vi "OTP - Determine bits.vi"(7 "Specification":T1={"Cmin (fF)"=500.0, "Cmin tolerance (%)"=10.0, "Cmax (fF)"=3460.0, "Cmax tolerance (%)"=1.38, "States"=32}, 8 "Cmax measured (fF)":dbl, 9 "Cmin measured (fF)":dbl=595.842, 10 "dCap (fF)":dbl[](array[numeric])=[216.58100000000002, 226.95699999999997, 198.55200000000005, 220.50100000000006, 199.26699999999997, 240.08200000000002, 67.724, 255.87100000000007, 215.32300000000004, 199.00000000000006, 230.48900000000006, 201.30599999999998, 137.042, 42.55399999999998], 11 "Register 2 & 3 (hex)":string[][](array[string])=[["1", "0"]]) -> (1 "Target values (fF)":dbl[](array[numeric]), 2 "Measured values (fF)":dbl[](array[numeric]), 3 "Register 2 & 3 (hex)":string[][](array[string]))   [LabVIEW 2020]
panel:
  out "Error":dbl[](graph)
  out "Measured vs. Target error (%)":dbl[](array[numeric])
  out "System Waveform Graph":dbl[][](graph)
  out "max value":dbl
  out "min value":dbl
  out "Setting indices":dbl[](array[numeric])
  out "Setting beams":bool[][](array[boolean])
  out "Measured-Target (fF)":dbl[](array[numeric])
  out "All comb. meas (fF)":dbl[](array[numeric])
  out "Target step (fF)":dbl
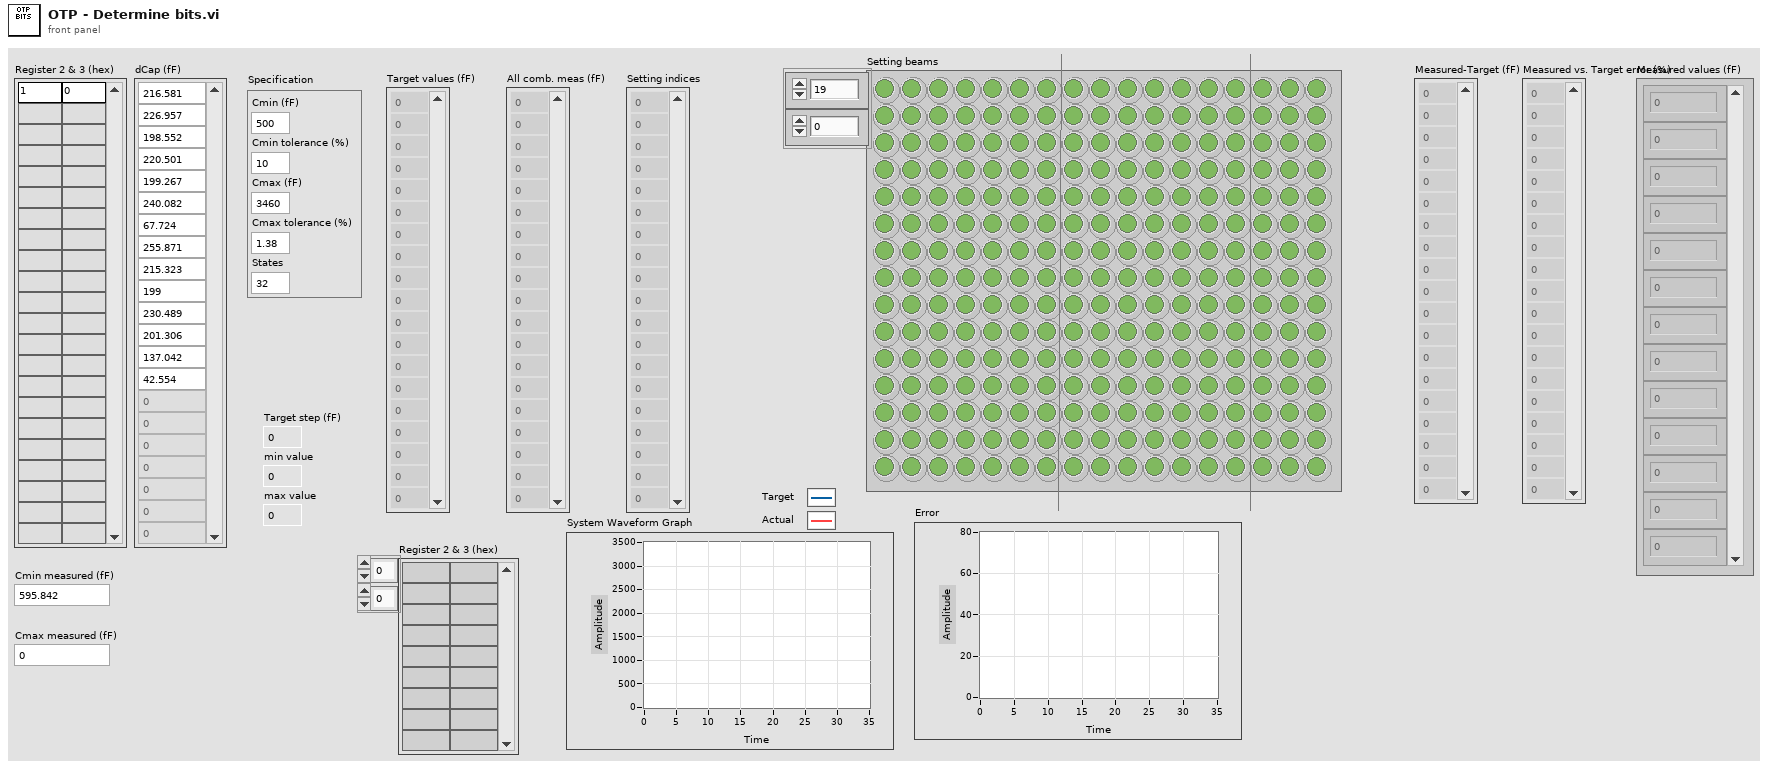
[diagram p1: front panel]
types:
  T1 = cluster{"Cmin (fF)":dbl, "Cmin tolerance (%)":dbl, "Cmax (fF)":dbl, "Cmax tolerance (%)":dbl, "States":i32}
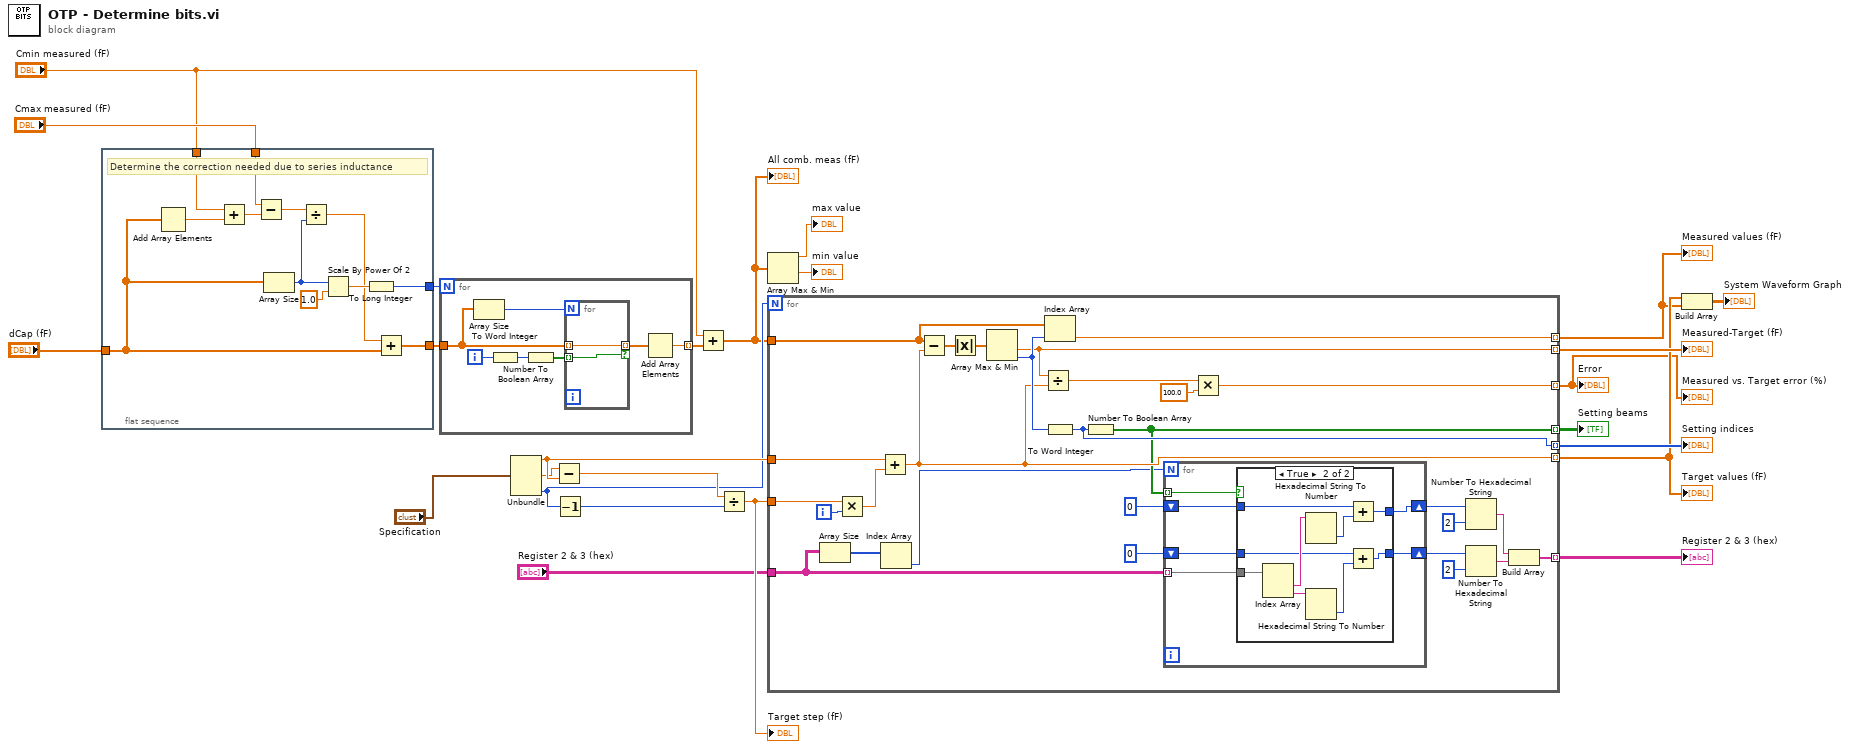
[diagram p0: block diagram]
diagram:
  n1 = flat-sequence {
    tunnel: "Cmax measured (fF)" -> [w36]
    tunnel: [w32] -> w5
    tunnel: "dCap (fF)" -> [w31]
    tunnel: [w30] -> w3
    tunnel: "Cmin measured (fF)" -> [w28]
    frame #0 {
      # "Determine the correction needed due to series inductance"
      n2 = Add Array Elements(numeric array=w31) -> (sum=w27:dbl)
      n3 = Add(x=w28, y=w27) -> (x+y=w26:dbl)
      n4 = Subtract(x=w36, y=w26) -> (x-y=w35:dbl)
      n5 = Array Size(array=w31) -> (size(s)=w34:i32)
      n6 = Divide(x=w35, y=w34) -> (x/y=w29:dbl)
      n7 = Scale By Power Of 2(n=w34, x=1.0) -> (x*2^n=w33:dbl)
      n8 = To Long Integer(number=w33) -> (32bit integer=w32:i32)
      n9 = Add(x=w29, y=w31) -> (x+y=w30:dbl[])
    }
  }
  n10 = for {
    N: w5 -> [_]
    tunnel: w3 -> [w41]
    tunnel: [w38] -> w22 mode=indexing
    i -> [w44]
    n11 = Array Size(array=w41) -> (size(s)=w40:i32)
    n12 = To Word Integer(number=w44) -> (16bit integer=w43:i16)
    n13 = Number To Boolean Array(number=w43) -> (Boolean array=w42:bool[])
    n14 = for {
      N: w40 -> [_]
      tunnel: w41 -> [w46] mode=indexing
      tunnel: w42 -> [w45] mode=indexing
      tunnel: [w46] -> w39 mode=indexing if=w45
    }
    n15 = Add Array Elements(numeric array=w39) -> (sum=w38:dbl)
  }
  n16 = Unbundle("Specification") -> ("Cmin (fF)"=w11:dbl, "Cmax (fF)"=w10:dbl, "States"=w9:i32)  [unwired: 2 out]
  n17 = Subtract(x=w10, y=w11) -> (x-y=w25:dbl)
  n18 = Decrement(x=w9) -> (x-1=w24:i32)
  n19 = Add(x="Cmin measured (fF)", y=w22) -> (x+y=w6:dbl[])
  "All comb. meas (fF)" <- w6
  n20 = Divide(x=w25, y=w24) -> (x/y=w23:dbl)
  "Target step (fF)" <- w23
  n21 = Array Max & Min(array=w6) -> (max value=→"max value":dbl, min value=→"min value":dbl)  [unwired: 2 out]
  n22 = for {
    N: w9 -> [_]
    tunnel: w11 -> [w72]
    tunnel: w23 -> [w71]
    tunnel: [w63] -> w16 mode=indexing
    tunnel: w6 -> [w66]
    tunnel: [w64] -> w21 mode=indexing
    tunnel: [w59] -> w20 mode=indexing
    tunnel: [w68] -> w19 mode=indexing
    tunnel: [w65] -> w15 mode=indexing
    tunnel: [w60] -> w8 mode=indexing
    tunnel: "Register 2 & 3 (hex)" -> [w58]
    tunnel: [w49] -> w13 mode=indexing
    i -> [w74]
    n23 = Array Size(array=w58) -> (size(s)=w57:i32[])
    n24 = Multiply(x=w71, y=w74) -> (x*y=w73:dbl)
    n25 = Add(x=w72, y=w73) -> (x+y=w63:dbl)
    n26 = Index Array(array=w57) -> (element=w56:i32)  [unwired: 1 in]
    n27 = Subtract(x=w66, y=w63) -> (x-y=w70:dbl[])
    n28 = Absolute Value(x=w70) -> (abs(x)=w69:dbl[])
    n29 = Array Max & Min(array=w69) -> (min value=w64:dbl, min index (indices)=w67:i32)  [unwired: 2 out]
    n30 = Divide(x=w64, y=w63) -> (x/y=w62:dbl)
    n31 = Index Array(array=w66, index=w67) -> (element=w65:dbl)
    n32 = To Word Integer(number=w67) -> (16bit integer=w68:i16)
    n33 = Number To Boolean Array(number=w68) -> (Boolean array=w59:bool[])
    n34 = for {
      N: w56 -> [_]
      tunnel: w58 -> [w80] mode=indexing
      tunnel: w59 -> [w79] mode=indexing
      shift-right: [w76] -> w53
      shift-left: u32 0 -> [w77]
      shift-right: [w75] -> w52
      shift-left: u32 0 -> [w78]
      n35 = case shown="True" w79 {
        tunnel: w80 -> [_ w91]
        tunnel: w78 -> [w81 w88]
        tunnel: w77 -> [w82 w85]
        tunnel: [w82 w83] -> w76
        tunnel: [w81 w87] -> w75
        frame False {
        }
        frame True {
          n36 = Index Array(array=w91) -> (element #1=w90:string, element #2=w89:string)  [unwired: 2 in]
          n37 = Hexadecimal String To Number(string=w90) -> (number=w86:u32)  [unwired: 2 in, 1 out]
          n38 = Hexadecimal String To Number(string=w89) -> (number=w84:u32)  [unwired: 2 in, 1 out]
          n39 = Add(x=w88, y=w86) -> (x+y=w87:u32)
          n40 = Add(x=w85, y=w84) -> (x+y=w83:u32)
        }
      }
    }
    n41 = Multiply(x=w62, y=100.0) -> (x*y=w60:dbl)
    n42 = Number To Hexadecimal String(1:i16 2 ("width (-)"), 2:w52) -> (0:w50:string)
    n43 = Number To Hexadecimal String(1:i16 2 ("width (-)"), 2:w53) -> (0:w51:string)
    n44 = Build Array(w50, w51) -> (w49:string[])
  }
  "Target values (fF)" <- w16
  "Measured-Target (fF)" <- w21
  "Setting beams" <- w20
  "Setting indices" <- w19
  "Measured values (fF)" <- w15
  "Measured vs. Target error (%)" <- w8
  "Register 2 & 3 (hex)" <- w13
  "Error" <- w8
  n45 = Build Array(w16, w15) -> (→"System Waveform Graph":dbl[][])
